vi "Get Measure.vi"(8 "error in (no error)":errorcluster caption="entrée d'erreur (pas d'erreur)", 11 "Class Multimeter Rigol DM3058 en entrée":refnum<class "Class Multimeter Rigol DM3058.lvclass">) -> (0 "error out":errorcluster caption="sortie d'erreur", 2 "Voltage":dbl, 3 "Class Multimeter Rigol DM3058 en sortie":refnum<class "Class Multimeter Rigol DM3058.lvclass">)   [LabVIEW 2020, in "Library Instrument & Equipement.lvlib" / "Library Multimeter.lvlib" / "Class Multimeter Rigol DM3058.lvclass"]
uses:
  Class Multimeter Rigol DM3058.lvclass
  C:/Users/ngarcin/OneDrive - Altyor/Standard TB/Class/Multimeter/Multimeter (Default)/Class Multimeter (Default).lvclass
  Class Multimeter Rigol DM3058.lvclass/Class Multimeter Rigol DM3058.ctl
  RIGOL DM3058/RIGOL DM3058.lvlib
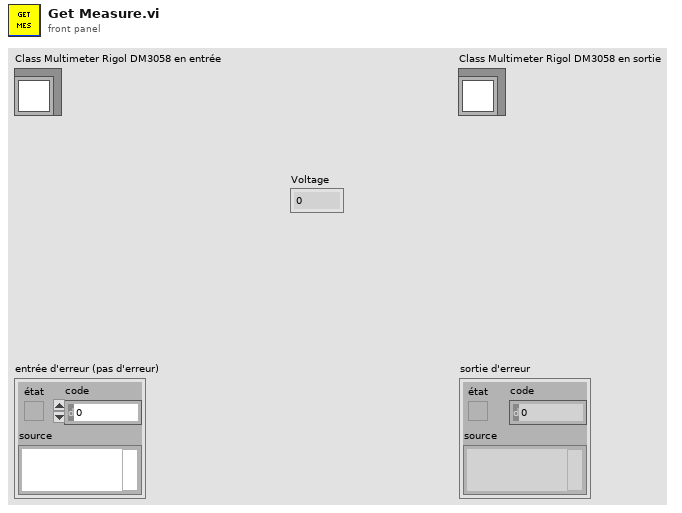
[diagram p1: front panel]
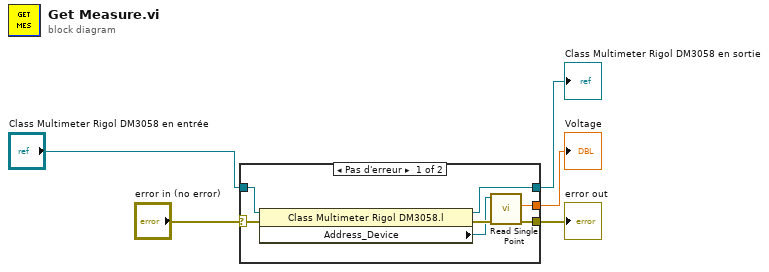
[diagram p0: block diagram]
diagram:
  n1 = case shown="Pas d'erreur" "error in (no error)" {
    selector: "error in (no error)" -> [w8 w14]
    tunnel: [w7 w14] -> w2
    tunnel: [w9 w13] -> w1
    tunnel: "Class Multimeter Rigol DM3058 en entrée" -> [w10 w13]
    tunnel: [w6 _] -> w3
    frame No Error {
      n2 = property class="Class Multimeter Rigol DM3058.l"(reference=w10, error in=w8) -> (reference out=w9:refnum<class "Class Multimeter Rigol DM3058.lvclass">, error out=w12:errorcluster, "Address_Device"=w11:refnum<visa-resource-name>)
      n3 = call "Read Single Point.vi"("error in (no error)"=w12, "VISA resource name"=w11) -> ("error out"=w7:errorcluster, "Measurement"=w6:dbl)  [unwired: 7 in, 1 out]
    }
    frame Error {
    }
  }
  "error out" <- w2
  "Class Multimeter Rigol DM3058 en sortie" <- w1
  "Voltage" <- w3
